vi "ChangeToDACcodes+CheckLimit.vi"(11 "Input Waveform":dbl[](array[numeric])) -> (3 "DAC Codes":u16[](array[numeric]))   [LabVIEW 2020]
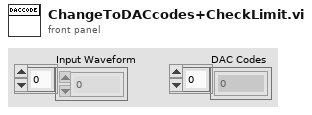
[diagram p1: front panel]
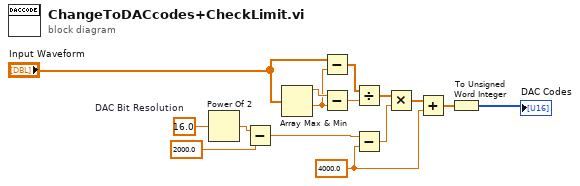
[diagram p0: block diagram]
diagram:
  w7 = 4000.0 ("y")
  w11 = 16.0  # DAC Bit Resolution
  n1 = Power Of 2(x=w11) -> (2^x=w3:dbl)
  n2 = Subtract(x=w3, y=2000.0) -> (x-y=w2:dbl)
  n3 = Array Max & Min(array="Input Waveform") -> (max value=w15:dbl, min value=w14:dbl)  [unwired: 2 out]
  n4 = Subtract(x="Input Waveform", y=w14) -> (x-y=w13:dbl[])
  n5 = Subtract(x=w15, y=w14) -> (x-y=w12:dbl)
  n6 = Divide(x=w13, y=w12) -> (x/y=w10:dbl[])
  n7 = Subtract(x=w2, y=w7) -> (x-y=w9:dbl)
  n8 = Multiply(x=w10, y=w9) -> (x*y=w8:dbl[])
  n9 = Add(x=w8, y=w7) -> (x+y=w6:dbl[])
  n10 = To Unsigned Word Integer(number=w6) -> (unsigned 16bit integer=→"DAC Codes":u16[])
